vi "ModelCode_Rf2.vi"(9 "BarCode":string, 11 "Data In":T1) -> (1 "ModeCode":string, 3 "Data Out":T1)   [LabVIEW 2014]
uses:
  controls/Data.ctl
panel:
  # "日期"
  # "機種名稱"
  # "機種代號"
  # "商品條碼"
  # "台"
  # "OK"
  # "NG"
  # "台"
  # "總計"
  # "台"
  # "日期"
  # "機種名稱"
  # "機種代號"
  # "商品條碼"
  # "台"
  # "OK"
  # "NG"
  # "台"
  # "總計"
  # "台"
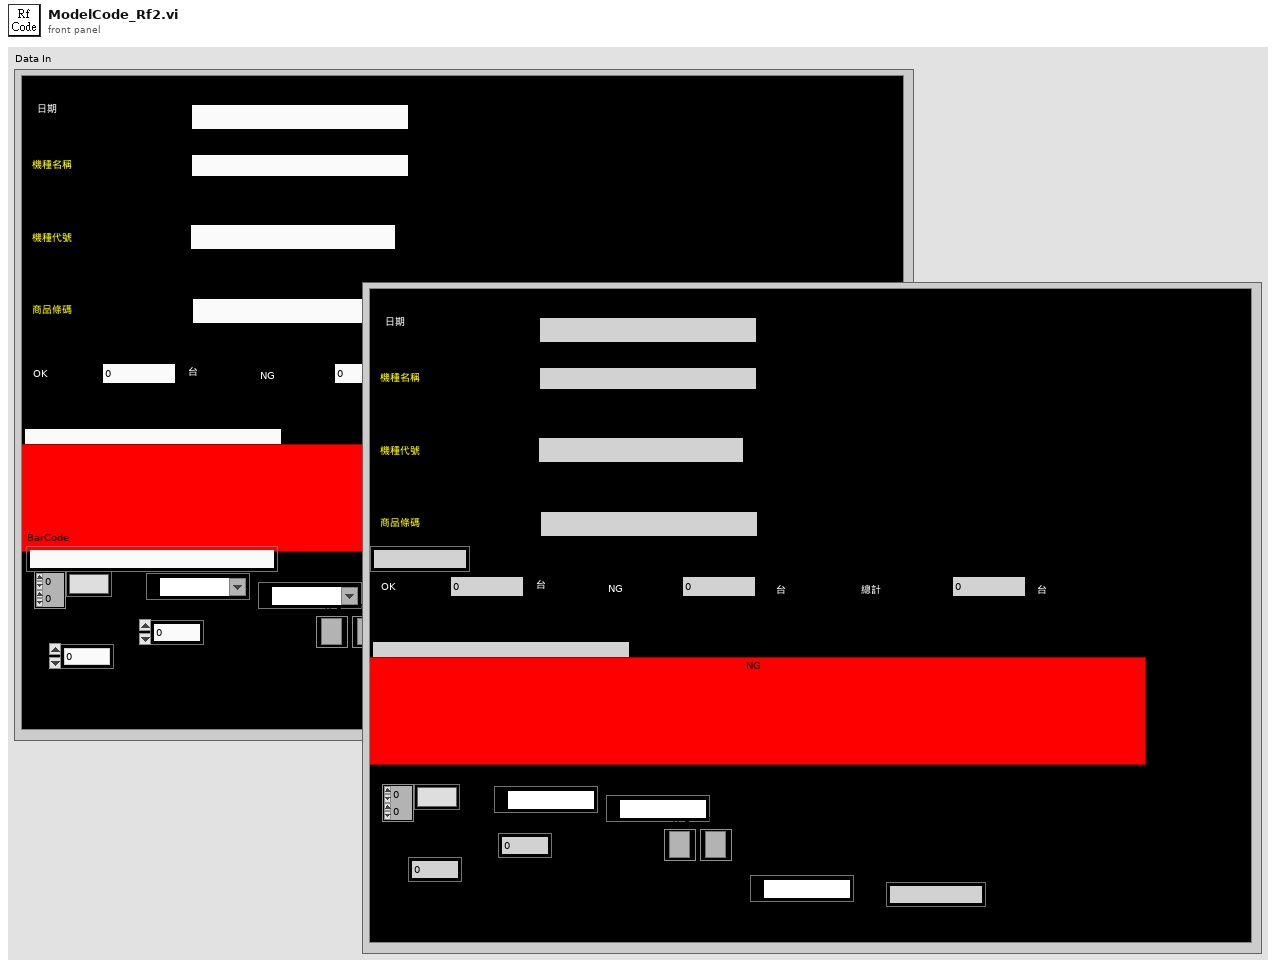
[diagram p1: front panel]
types:
  T1 = typedef "Data.ctl" = cluster{"Date":string, "BarCode1":string, "BarCode2":string, "BarCode3":string, "Message":string, "OK Count":u16, "NG Count":u16, "Total Count":u16, "ModelData":string[][], "OK&NG":bool, "COM1":refnum<visa-resource-name>, "COM2":refnum<visa-resource-name>, "IO":i32, "Time":u32, "TCP":refnum<k5>, "TCP 2":refnum<k5>, "COM3":refnum<visa-resource-name>, "CheckPars":string}
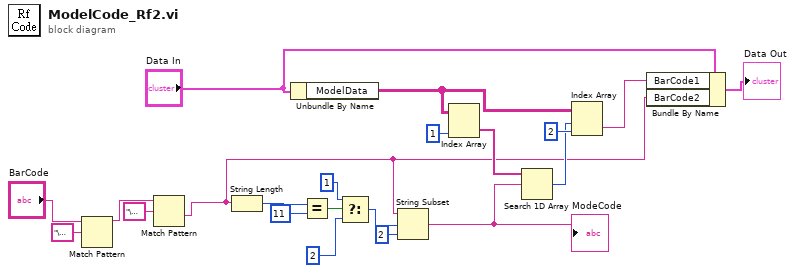
[diagram p0: block diagram]
diagram:
  n1 = Match Pattern(string="BarCode", regular expression="\u0003") -> (before substring=w3:string)  [unwired: 1 in, 3 out]
  n2 = Match Pattern(string=w3, regular expression="\u0002") -> (after substring=w1:string)  [unwired: 1 in, 3 out]
  n3 = String Length(string=w1) -> (length=w21:i32)
  n4 = Unbundle By Name("Data In") -> ("ModelData"=w11:string[][])
  n5 = Equal?(x=w21, y=11) -> (x = y?=w19:bool)
  n6 = Select(t=1 ("offset (0)"), s=w19, f=2) -> (s? t:f=w17:i32)
  n7 = String Subset(string=w1, offset (0)=w17, length (rest)=2 ("length (rest)")) -> (substring=w12:string)
  "ModeCode" <- w12
  n8 = Index Array(array=w11, index (col)=1 ("disabled index (col)")) -> (element=w13:string[])  [unwired: 1 in]
  n9 = Search 1D Array(1D array=w13, element=w12) -> (index of element=w9:i32)  [unwired: 1 in]
  n10 = Index Array(array=w11, index (row)=w9, index (col)=2 ("disabled index (col)")) -> (element=w6:string)
  n11 = Bundle By Name(cluster="Data In", "BarCode1"=w6, "BarCode2"=w1) -> (→"Data Out":T1)
